vi "Run TopLevel Several Times.vi"() -> ()   [LabVIEW 2013]
uses:
  Controls/Problem Instance Type.ctl
  Classes/GA_Class/Controls/Crossover Type.ctl
  Classes/GA_Class/Controls/Mutation Type.ctl
  Controls/Local Search Type.ctl
  Classes/SA_Class/Controls/Perturbation Method.ctl
  Classes/GA.lvclass
  Classes/SA.lvclass
panel:
  in  "Perturbation Method For SA":T1
  in  "Local Search":T2
  in  "Mutation Type":T3
  in  "Crossover Type":T4=enum."Linear Order Cx (LOX)"
  in  "Number Of Runs":i32=5
  in  "Instance Number":dbl format="%#_13g"
  in  "Instance Type":T5=enum."Brucker"
  in  "file path (use dialog)":path=path "C:/Users/Alper/Desktop/Tez/LabVIEWProjects/OSSP_Project/instances/Openshop_Instances/brucker/j3-per10-0.txt"
  out "Results":u16[](array[numeric])=[862, 970, 961, 900, 1022]
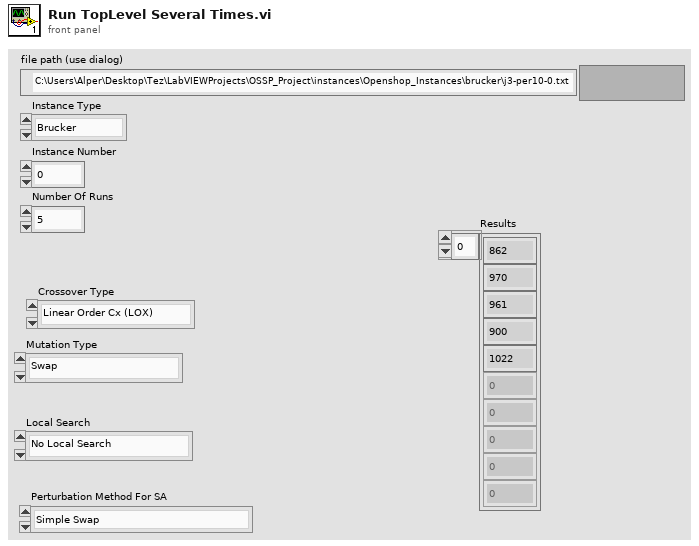
[diagram p1: front panel]
types:
  T1 = typedef "SA.lvclass/Perturbation Method.ctl" = enum16{"Simple Swap", "Insert", "NonRedundantSwap", "Job Order Swap", "Machine Order Swap", "Machine&Job Order Swap", "Critical Path Swap"}
  T2 = typedef "Local Search Type.ctl" = enum16{"No Local Search", "SA Population", "IRH3T(Pop)", "IRH3T(Best Solution)", "SA Best Solution", "SA Random Solution", "SA Random 3 Solutions", "SA Hybrid", "VNS Best Solution", "VNS Random Solution"}
  T3 = typedef "GA.lvclass/Mutation Type.ctl" = enum16{"Swap", "Non-Redundant Swap", "Insert", "Shift", "Shuflle", "Inversion", "SA", "IRH3T", "JO4M Swap", "MO4J Swap", "SPT JO4M", "LCTJ Swap", "Low's Mutation", "ND Mutation"}
  T4 = typedef "GA.lvclass/Crossover Type.ctl" = enum16{"One Point Cx", "Two Point Cx", "Ordered Cx (OX)", "Linear Order Cx (LOX)", "Cycle Cx", "Specialized Cx", "JO4M Cx", "MPOX1", "MPOX1 Random", "MPOX2", "MPOX2 Random"}
  T5 = typedef "Problem Instance Type.ctl" = enum16{"Taillard", "Gueret-Prins", "Brucker"}
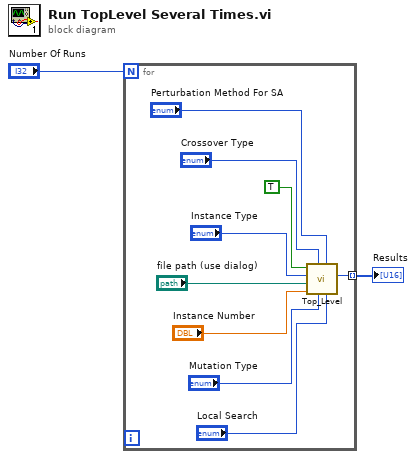
[diagram p0: block diagram]
diagram:
  n1 = for {
    N: "Number Of Runs" -> [_]
    tunnel: [w9] -> w2 mode=indexing
    n2 = call "Top_Level.vi"("Local Search"="Local Search", "Perturbation Method"="Perturbation Method For SA", "Mutation Type"="Mutation Type", "Crossover Type"="Crossover Type", "Instance Number"="Instance Number", "file path (use dialog)"="file path (use dialog)", "Instance Type"="Instance Type", "Auto Mode"=TRUE) -> ("Result"=w9:u16)  [unwired: 3 in]
  }
  "Results" <- w2
